vi "h.ACQ.ParseSensorsHeader.vi"(11 "Header from #GetPeaks":u8[](array[numeric])) -> (0 "Status":u8, 1 "Time Stamp (ns)":u64, 2 "SN":u64, 3 "Header Length":u16)   [LabVIEW 2016, in "h.Library.lvlib"]
doc: "This vi parses the header returned by the #GetPeaks command and returns the contained data through a number of outputs.\n\n<b>Header from #GetPeaks</b> - data returned by #GetPeaks.vi\n<b>Header Version</b> - Version number of the header\n<b>Header Length</b> - The total header length in bytes (also the start of the peaks data)s\n<b>SN</b> - Serial Number of the collected data set\n<b>Time Stamp</b> - The estimated time in ns when the instrument acquired the spectrum\n<b>#Peaks</b> - Array containing the number of detected peaks on each channel"
uses:
  h.Library.lvlib
panel:
  out "Reserved2":u32
  out "Reserved1":u32
  out "Buffer Percentage":u8
  # "Hyperion Parse Sensors Header"
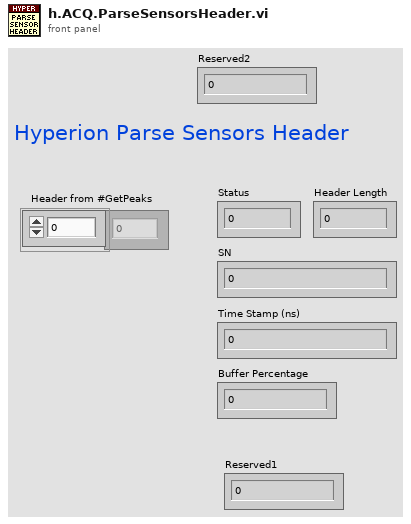
[diagram p1: front panel]
types:
  T1 = enum16{"big-endian, network order", "native, host order", "little-endian"}
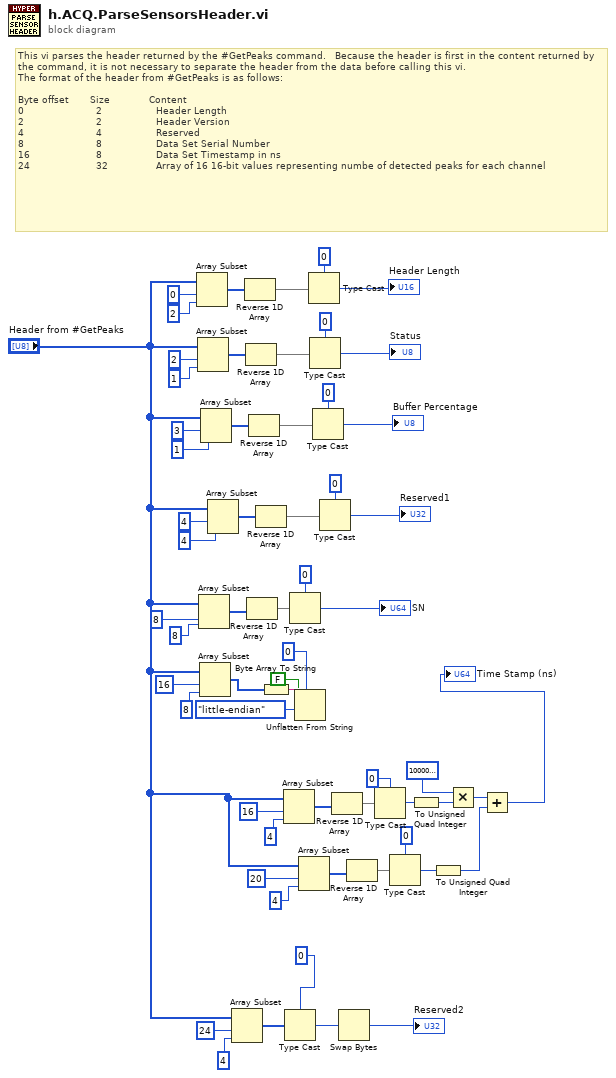
[diagram p0: block diagram]
diagram:
  # "This vi parses the header returned by the #GetPeaks command.   Because the header is first in the content returned by the command, it is not necessary to separate the header from the data before calling this vi.\nThe format of the header from #GetPeaks is as follows:\n\nByte offset       Size             Content\n0                        2                  Header Length\n2                        2                  Header Version\n4                        4                  Reserved\n8                        8                  Data Set Serial Number\n16                      8                  Data Set Timestamp in ns\n24                      32                Array of 16 16-bit values representing numbe of detected peaks for each channel"
  n1 = Array Subset(array="Header from #GetPeaks", index=0, length=2) -> (w41:u8[])
  n2 = Array Subset(array="Header from #GetPeaks", index=2, length=1) -> (w55:u8[])
  n3 = Array Subset(array="Header from #GetPeaks", index=8, length=8) -> (w50:u8[])
  n4 = Array Subset(array="Header from #GetPeaks", index=16, length=8) -> (w23:u8[])
  n5 = Array Subset(array="Header from #GetPeaks", index=3, length=1) -> (w34:u8[])
  n6 = Array Subset(array="Header from #GetPeaks", index=4, length=4) -> (w29:u8[])
  n7 = Array Subset(array="Header from #GetPeaks", index=24, length=4 ("y")) -> (w38:u8[])
  n8 = Reverse 1D Array(array=w41) -> (reversed array=w42:u8[])
  n9 = Reverse 1D Array(array=w55) -> (reversed array=w56:u8[])
  n10 = Reverse 1D Array(array=w50) -> (reversed array=w49:u8[])
  n11 = Reverse 1D Array(array=w34) -> (reversed array=w35:u8[])
  n12 = Reverse 1D Array(array=w29) -> (reversed array=w28:u8[])
  n13 = Byte Array To String(unsigned byte array=w23) -> (string=w22:string)
  n14 = Array Subset(array="Header from #GetPeaks", index=16, length=4) -> (w5:u8[])
  n15 = Type Cast(type=u32 0 ("length"), x=w38) -> (*(type *) &x=w60:u32)
  n16 = Type Cast(type=u64 0 ("length"), x=w49) -> (*(type *) &x=→"SN":u64)
  n17 = Unflatten From String(type=u64 0 ("length"), binary string=w22, data includes array or string size? (T)=FALSE, byte order (0:big-endian, network order)=T1."little-endian") -> ()  [unwired: 1 in, 3 out]
  n18 = Array Subset(array="Header from #GetPeaks", index=20, length=4) -> (w16:u8[])
  n19 = Type Cast(type=u16 0 ("length"), x=w42) -> (*(type *) &x=→"Header Length":u16)
  n20 = Type Cast(type=u8 0 ("length"), x=w56) -> (*(type *) &x=→"Status":u8)
  n21 = Type Cast(type=u8 0 ("length"), x=w35) -> (*(type *) &x=→"Buffer Percentage":u8)
  n22 = Type Cast(type=u32 0 ("length"), x=w28) -> (*(type *) &x=→"Reserved1":u32)
  n23 = Reverse 1D Array(array=w5) -> (reversed array=w6:u8[])
  n24 = Swap Bytes(anything=w60) -> (byte swapped=→"Reserved2":u32)
  n25 = Reverse 1D Array(array=w16) -> (reversed array=w10:u8[])
  n26 = Type Cast(type=u32 0 ("length"), x=w6) -> (*(type *) &x=w15:u32)
  n27 = Type Cast(type=u32 0 ("length"), x=w10) -> (*(type *) &x=w14:u32)
  n28 = To Unsigned Quad Integer(1:w15) -> (0:w17:u64)
  n29 = To Unsigned Quad Integer(1:w14) -> (0:w13:u64)
  n30 = Multiply(x=u64 1000000000 ("y"), y=w17) -> (x*y=w12:u64)
  n31 = Add(x=w12, y=w13) -> (x+y=→"Time Stamp (ns)":u64)
